vi "Fan Read-Write.vi"(0 "Hellicopter Tasks Input":T1, 7 "Fan Input":dbl, 11 "Error In":errorcluster) -> (4 "Hellicopter Tasks Output":T1, 8 "L/C Output":dbl, 15 "Error Out":errorcluster)   [LabVIEW 2017]
uses:
  <vilib>/DAQmx/read.llb/DAQmx Read (Analog 2D DBL NChan NSamp).vi
  <vilib>/DAQmx/read.llb/DAQmx Read (Counter DBL 1Chan 1Samp).vi
  <vilib>/DAQmx/write.llb/DAQmx Write (Analog 1D DBL NChan 1Samp).vi
  <vilib>/DAQmx/write.llb/DAQmx Write (Digital 1D Bool NChan 1Samp 1Line).vi
  <vilib>/Analysis/baseanly.llb/Mean (DBL).vi
  <vilib>/DAQmx/miscellaneous.llb/DAQmx Fill In Error Info.vi
  <vilib>/Analysis/NI_AALBase.lvlib
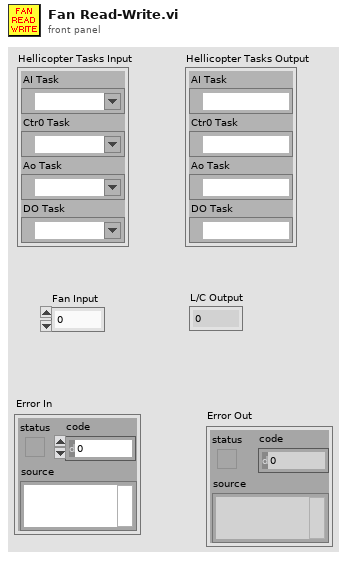
[diagram p1: front panel]
types:
  T1 = cluster{"AI Task":refnum<k21>, "Ctr0 Task":refnum<k21>, "Ao Task":refnum<k21>, "DO Task":refnum<k21>}
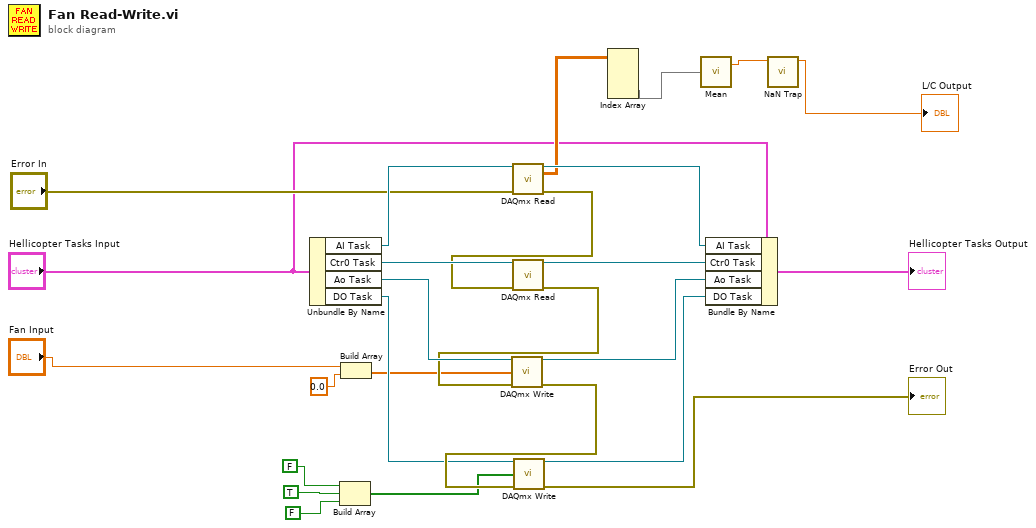
[diagram p0: block diagram]
diagram:
  n1 = Unbundle By Name("Hellicopter Tasks Input") -> ("AI Task"=w23:refnum<k21>, "Ctr0 Task"=w21:refnum<k21>, "Ao Task"=w22:refnum<k21>, "DO Task"=w12:refnum<k21>)
  n2 = Build Array(FALSE, TRUE ("element"), FALSE ("element")) -> (w10:bool[])
  n3 = Build Array("Fan Input", 0.0 ("element")) -> (w6:dbl[])
  n4 = call-poly <vilib>:"DAQmx Read.vi"("task/channels in"=w23, "error in"="Error In") -> ("task out"=w26:refnum<k21>, "data"=w17:dbl[][], "error out"=w20:errorcluster)  [unwired: 11 in]
  n5 = call-poly <vilib>:"DAQmx Read.vi"("task/channels in"=w21, "error in"=w20) -> ("task out"=w25:refnum<k21>, "error out"=w19:errorcluster)  [unwired: 11 in, 1 out]
  n6 = call-poly <vilib>:"DAQmx Write.vi"("task/channels in"=w22, "data"=w6, "error in"=w19) -> ("task out"=w24:refnum<k21>, "error out"=w16:errorcluster)  [unwired: 10 in, 1 out]
  n7 = call-poly <vilib>:"DAQmx Write.vi"("task/channels in"=w12, "data"=w10, "error in"=w16) -> ("task out"=w11:refnum<k21>, "error out"=→"Error Out":errorcluster)  [unwired: 10 in, 1 out]
  n8 = Index Array(array=w17) -> (element #2=w5:dbl[])  [unwired: 4 in, 1 out]
  n9 = call-poly <vilib>:"Mean.vi"("X"=w5) -> ("mean"=w4:dbl)  [unwired: 1 out]
  n10 = Bundle By Name(cluster="Hellicopter Tasks Input", "AI Task"=w26, "Ctr0 Task"=w25, "Ao Task"=w24, "DO Task"=w11) -> (→"Hellicopter Tasks Output":T1)
  n11 = call "NaN Trap.vi"("Elevation in"=w4) -> ("Elevation out"=→"L/C Output":dbl)  [unwired: 9 in, 1 out]
